vi "ClimbExtend.vi"(11 "Button":bool) -> (3 "Complete?":bool)   [LabVIEW 2015]
panel:
  in  "Motor Power":dbl
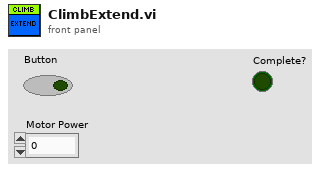
[diagram p1: front panel]
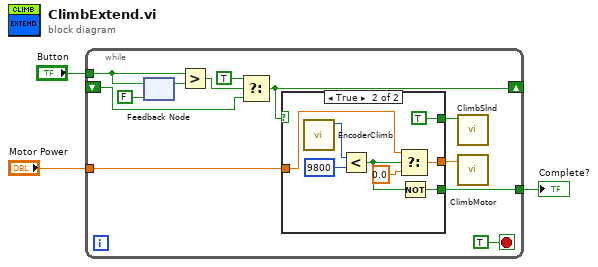
[diagram p0: block diagram]
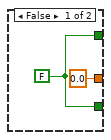
[diagram p2: hidden frame]
diagram:
  n1 = while {
    tunnel: "Button" -> [w14]
    shift-right: [w12] -> _
    shift-left: _ -> [w13]
    tunnel: [w5] -> w2
    tunnel: "Motor Power" -> [w4]
    stop <- TRUE stop-if-true
    n2 = feedback #1(FALSE) -> (w9:bool)
    n3 = feedback-in #1(w14) -> ()
    n4 = Greater?(x=w14, y=w9) -> (0:w8:bool)
    n5 = Select(t=TRUE, s=w8, f=w13) -> (s? t:f=w12:bool)
    n6 = case shown="True" w12 {
      tunnel: [w16 TRUE] -> w11
      tunnel: [0.0 w21] -> w6
      tunnel: [w16 w20] -> w5
      tunnel: w4 -> [_ w18]
      frame False {
        w16 = FALSE
      }
      frame True {
        n7 = call "EncoderClimb.vi"() -> ("Position_out"=w25:i32)  [unwired: 11 in]
        n8 = Less?(x=w25, y=9800) -> (x < y?=w19:bool)
        n9 = Select(t=w18, s=w19, f=0.0) -> (s? t:f=w21:dbl)
        n10 = Not(x=w19) -> (.not. x?=w20:bool)
      }
    }
    n11 = call "ClimbSlnd.vi"("Button"=w11) -> ()  [unwired: 11 in]
    n12 = call "ClimbMotor.vi"("Power"=w6) -> ()  [unwired: 11 in]
  }
  "Complete?" <- w2
